vi "Test.vi"() -> ()   [LabVIEW 2011, in "Michell Easidew.lvclass"]
uses:
  Michell Easidew.lvclass
panel:
  out "Relative Humidity":dbl
  out "error out":errorcluster={"status"=FALSE, "code"=1073676294, "source"="VISA Read in Michell Easydew.lvclass:Get Dew Point.vi->Michell Easydew.lvclass:Test.vi"}
  out "Michell Easydew out":refnum<class "Michell Easidew.lvclass">
  in  "stop":bool
  out "Dew Point":dbl=-36.4
  in  "Michell Easydew in":refnum<class "Michell Easidew.lvclass">
  in  "error in":errorcluster
  in  "VISA resource name":refnum<visa-resource-name>="COM6"
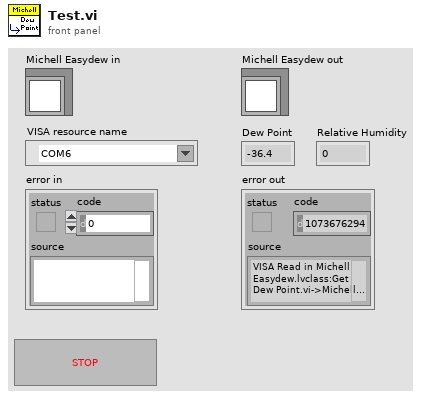
[diagram p1: front panel]
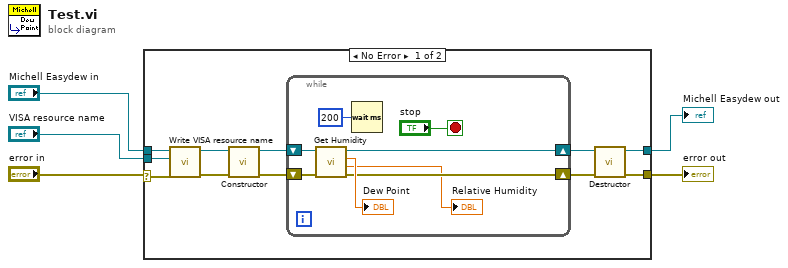
[diagram p0: block diagram]
diagram:
  n1 = case shown="No Error" "error in" {
    selector: "error in" -> [w6 w25]
    tunnel: "Michell Easydew in" -> [w16 w26]
    tunnel: "VISA resource name" -> [w15 _]
    tunnel: [w8 w26] -> w3
    tunnel: [w7 w25] -> w2
    frame No Error {
      n2 = call-dynamic "Write VISA resource name.vi"("error in (no error)"=w6, "VISA resource name"=w15, "Michell Easydew in"=w16) -> ("error out"=w14:errorcluster, "Michell Easydew out"=w13:refnum<class "Michell Easidew.lvclass">)  [unwired: 7 in]
      n3 = call-dynamic "Constructor.vi"("error in (no error)"=w14, "Michell Easydew in"=w13) -> ("error out"=w12:errorcluster, "Michell Easydew out"=w11:refnum<class "Michell Easidew.lvclass">)  [unwired: 8 in]
      n4 = while {
        shift-right: [w18] -> w9
        shift-left: w12 -> [w23]
        shift-right: [w19] -> w10
        shift-left: w11 -> [w24]
        stop <- "stop" stop-if-true
        n5 = call-dynamic "Get Humidity.vi"("error in"=w23, "Michell Easydew in"=w24) -> ("error out"=w18:errorcluster, "Relative Humidity"=→"Relative Humidity":dbl, "Dew Point"=→"Dew Point":dbl, "Michell Easydew out"=w19:refnum<class "Michell Easidew.lvclass">)  [unwired: 4 in, 2 out]
        n6 = Wait (ms)(milliseconds to wait=u32 200) -> ()  [unwired: 1 out]
      }
      n7 = call-dynamic "Destructor.vi"("error in"=w9, "Michell Easydew in"=w10) -> ("error out"=w7:errorcluster, "Michell Easydew out"=w8:refnum<class "Michell Easidew.lvclass">)  [unwired: 8 in]
    }
    frame Error {
    }
  }
  "Michell Easydew out" <- w3
  "error out" <- w2
